vi "build_client.vi"(5 "Client type":refnum<class "Client.lvclass">, 8 "error in (no error)":errorcluster, 11 "ClientBuilder in":refnum<class "ClientBuilder.lvclass">) -> (0 "error out":errorcluster, 2 "Client out":refnum<class "Client.lvclass">)   [LabVIEW 2020, in "reqwest.lvlib" / "ClientBuilder.lvclass"]
uses:
  ClientBuilder.lvclass
  Client/Client.lvclass
  ClientBuilder.lvclass/ClientBuilder.ctl
  lv_reqwest_64.dll
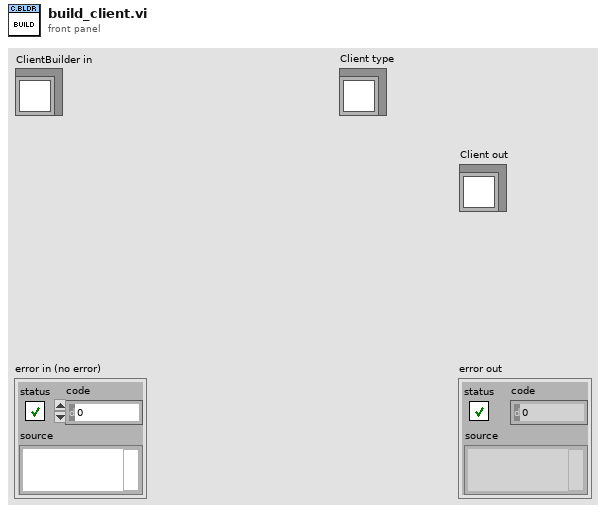
[diagram p1: front panel]
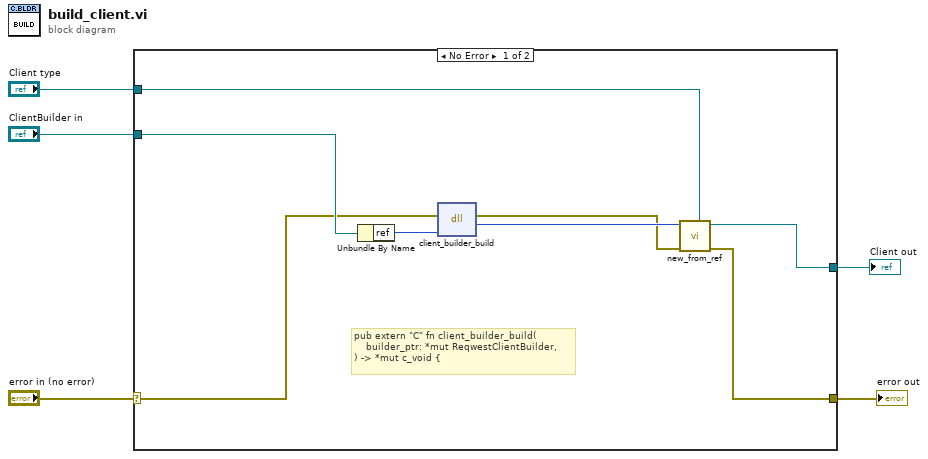
[diagram p0: block diagram]
diagram:
  n1 = case shown="No Error" "error in (no error)" {
    selector: "error in (no error)" -> [w11 w14]
    tunnel: "ClientBuilder in" -> [w12 _]
    tunnel: [w7 w14] -> w3
    tunnel: [w9 _] -> w2
    tunnel: "Client type" -> [w6 _]
    frame No Error {
      # "pub extern \"C\" fn client_builder_build(\n    builder_ptr: *mut ReqwestClientBuilder,\n) -> *mut c_void {"
      n2 = Unbundle By Name(w12) -> ("ref"=w13:u64)
      n3 = dll-call lib="C:/Projects/reqwest-rs-labview/lv_src/lv_reqwest_*.*" fn="client_builder_build"(error in=w11, "client_builder_ref"=w13) -> (error out=w8:errorcluster, "client_ref"=w10:u64)  [unwired: 3 in, 1 out]
      n4 = call "new_from_ref.vi"("Client in"=w6, "error in (no error)"=w8, "client_ref"=w10) -> ("error out"=w7:errorcluster, "Client out"=w9:refnum<class "Client.lvclass">)  [unwired: 7 in]
    }
    frame Error {
    }
  }
  "error out" <- w3
  "Client out" <- w2
